vi "Set Amplitude.vi"(11 "Amplitude":dbl) -> (0 "error out":errorcluster, 3 "Response":string)   [LabVIEW 2025, in "MCP Demo Application.lvlib"]
doc: "Sets the amplitude of the 3 channels."
uses:
  MCP Demo Application.lvlib
  Globals.vi
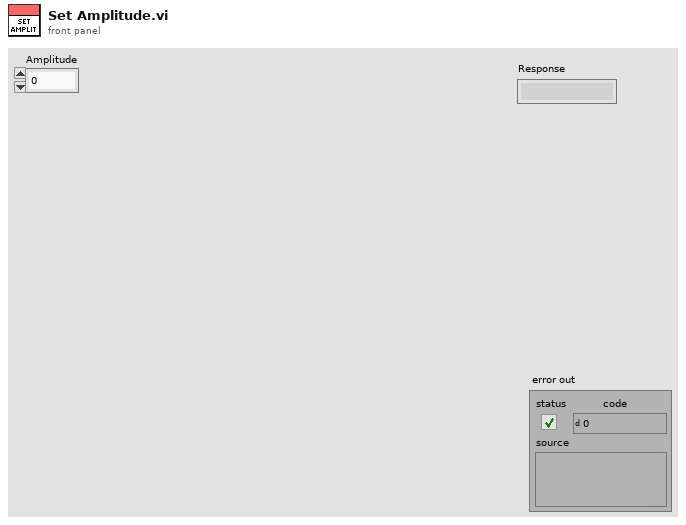
[diagram p1: front panel]
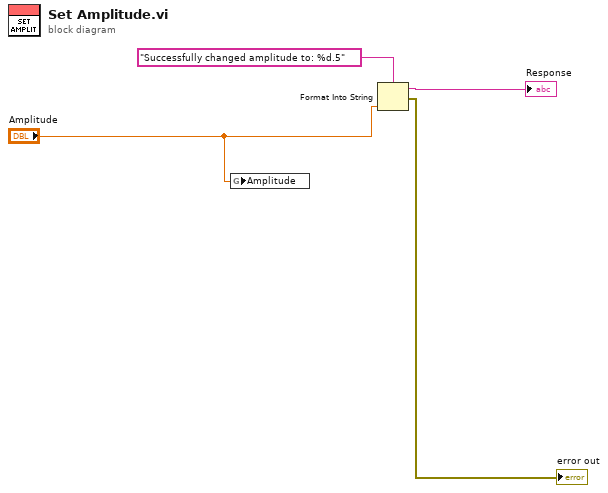
[diagram p0: block diagram]
diagram:
  n1 = global write "Globals.vi" "Amplitude"("Amplitude") -> ()
  n2 = Format Into String(format string="Successfully changed amplitude to: %d.5", "Amplitude") -> (resulting string=→"Response":string, error out=→"error out":errorcluster)  [unwired: 2 in]
